vi "disable offset.vi"(8 "error in (no error)":errorcluster, 11 "Thorcam in":refnum<class "Thorcam.lvclass">) -> (0 "error out":errorcluster, 1 "Value":i32, 3 "Thorcam out":refnum<class "Thorcam.lvclass">)   [LabVIEW 2012, in "Thorcam.lvclass"]
uses:
  Thorcam.lvclass
  Thorcam.lvclass/Thorcam.ctl
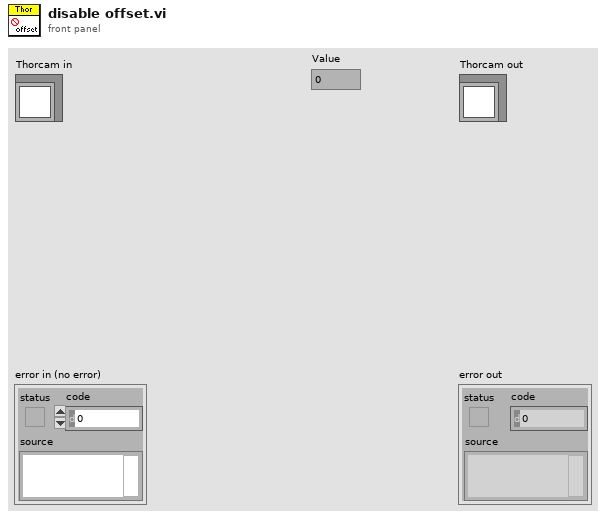
[diagram p1: front panel]
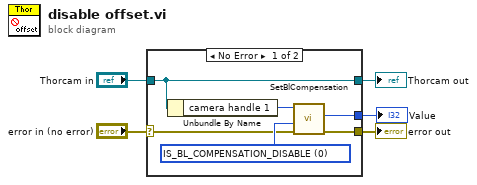
[diagram p0: block diagram]
diagram:
  n1 = case shown="No Error" "error in (no error)" {
    selector: "error in (no error)" -> [w8 w13]
    tunnel: [w7 w13] -> w4
    tunnel: [w9 w12] -> w2
    tunnel: "Thorcam in" -> [w9 w12]
    tunnel: [w6 _] -> w1
    frame No Error {
      w11 = 0 items=["IS_BL_COMPENSATION_DISABLE"=0, "IS_BL_COMPENSATION_ENABLE"=1, "IS_GET_BL_COMPENSATION"=32768, "IS_GET_BL_OFFSET"=32769, "IS_GET_BL_DEFAULT_MODE"=32770, "IS_GET_BL_DEFAULT_OFFSET"=32771, "IS_GET_BL_SUPPORTED_MODE"=32772, "IS_IGNORE_PARAMETER"=-1] ("Mode")
      n2 = Unbundle By Name(w9) -> ("camera handle 1"=w10:u32)
      n3 = call <instrlib>:"SetBlCompensation.vi"("error in"=w8, "Mode"=w11, "Camera Handle In"=w10) -> ("error out"=w7:errorcluster, "Value"=w6:i32)  [unwired: 6 in, 1 out]
    }
    frame Error {
    }
  }
  "error out" <- w4
  "Thorcam out" <- w2
  "Value" <- w1
